vi "invernadero.vi"() -> ()   [LabVIEW 2020]
panel:
  out "Humed.Actual":dbl
  out "Temp.Actual":dbl
  in  "Sistema":bool
  out "Waveform Chart":dbl(graph)
  out "Refrijeracion":bool
  out "Ventilacion":bool
  out "Regadera":bool
  out "Humedad\nInvernadero":dbl(knob) scale=0.0..100.0
  out "Temperatura\nInvernadero":dbl(slide) scale=0.0..100.0
  in  "Temperatura \nAmbiental":dbl(knob) scale=0.0..100.0
  in  "Humedad\nAmbiental":dbl(knob) scale=0.0..100.0
  in  "Humed.Min":dbl
  in  "Humed.Max":dbl
  in  "Temp.Min":dbl
  in  "Temp.Max":dbl
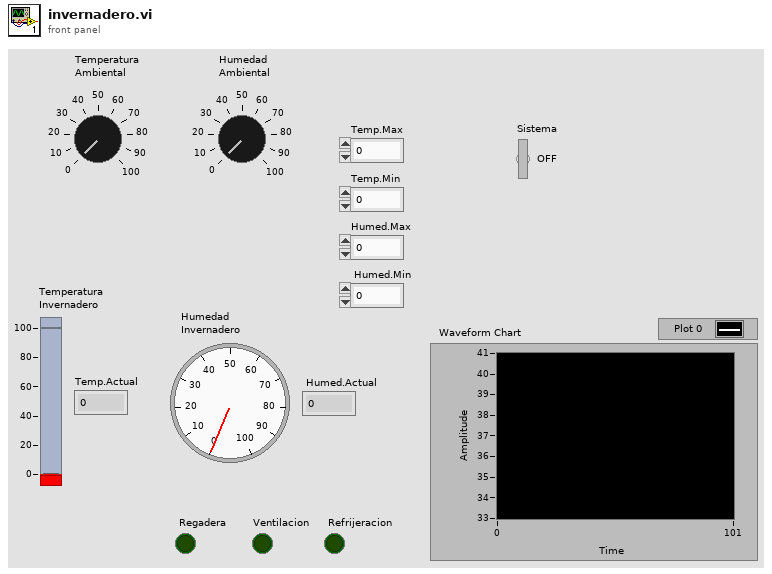
[diagram p1: front panel]
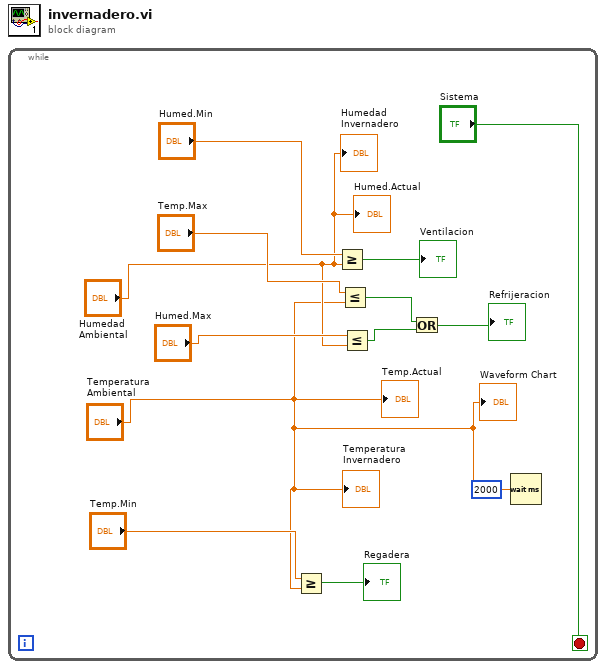
[diagram p0: block diagram]
diagram:
  n1 = while {
    stop <- "Sistema" stop-if-true
    (unwired) u32 2000 ("milliseconds to wait")
    n2 = Greater Or Equal?(x="Temp.Min", y="Temperatura \nAmbiental") -> (x >= y?=→"Regadera":bool)
    n3 = Greater Or Equal?(x="Humed.Min", y="Humedad\nAmbiental") -> (x >= y?=→"Ventilacion":bool)
    n4 = Less Or Equal?(x="Temp.Max", y="Temperatura \nAmbiental") -> (x <= y?=w12:bool)
    n5 = Less Or Equal?(x="Humed.Max", y="Humedad\nAmbiental") -> (x <= y?=w11:bool)
    n6 = Or(x=w12, y=w11) -> (x .or. y?=→"Refrijeracion":bool)
    n7 = Wait (ms)(milliseconds to wait="Temperatura \nAmbiental") -> ()  [unwired: 1 out]
    "Temperatura\nInvernadero" <- "Temperatura \nAmbiental"
    "Humedad\nInvernadero" <- "Humedad\nAmbiental"
    "Waveform Chart" <- "Temperatura \nAmbiental"
    "Temp.Actual" <- "Temperatura \nAmbiental"
    "Humed.Actual" <- "Humedad\nAmbiental"
  }
